vi "Get Protocol Type.vi"(8 "error in (no error)":errorcluster, 11 "RS-xxx to GPIB ConvBox in":refnum<class "RS-xxx to GPIB ConvBox.lvclass">) -> (0 "error out":errorcluster, 2 "protocol type":T1=enum."AK RS-XXX", 3 "RS-xxx to GPIB ConvBox out":refnum<class "RS-xxx to GPIB ConvBox.lvclass">)   [LabVIEW 2023, in "Protocols.lvlib" / "RS-xxx to GPIB ConvBox.lvclass"]
doc: "Returns GPIB ConvBox protocol type Enum."
uses:
  RS-xxx to GPIB ConvBox.lvclass
  Protocol Parent/Types/Protocol Type.ctl
  Protocol Parent/Protocol Parent.lvclass
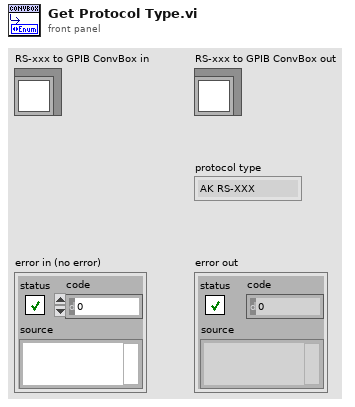
[diagram p1: front panel]
types:
  T1 = typedef "Protocols.lvlib/Protocol Parent.lvclass/Protocol Type.ctl" = enum16{"RS-XXX", "AK RS-XXX", "VISA", "TCPIP", "AK TCPIP", "UDP", "GPIB ConvBox"}
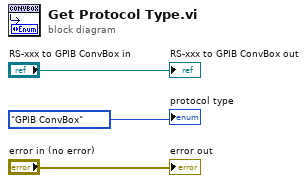
[diagram p0: block diagram]
diagram:
  "error out" <- "error in (no error)"
  "RS-xxx to GPIB ConvBox out" <- "RS-xxx to GPIB ConvBox in"
  "protocol type" <- Protocol_Type."GPIB ConvBox" ("Protocol out")
